vi "Extract zero offset.vi"(10 "Zero avg num":i32, 11 "Array":dbl[](array[numeric])) -> (3 "Offset":dbl)   [LabVIEW 2024]
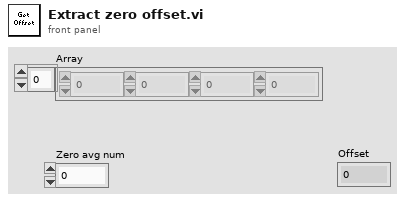
[diagram p1: front panel]
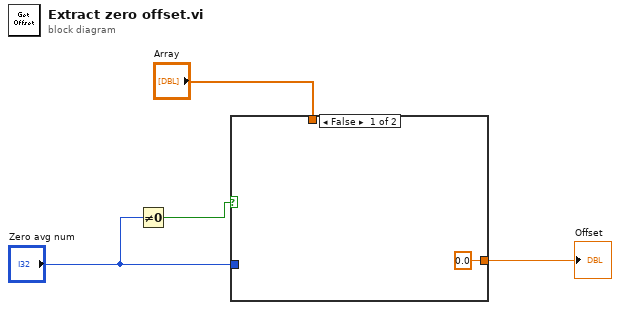
[diagram p0: block diagram]
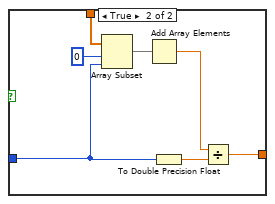
[diagram p2: hidden frame]
diagram:
  n1 = Not Equal To 0?(x="Zero avg num") -> (x != 0?=w1:bool)
  n2 = case shown="False" w1 {
    tunnel: "Array" -> [_ w12]
    tunnel: [0.0 w11] -> w3
    tunnel: "Zero avg num" -> [_ w9]
    frame False {
    }
    frame True {
      n3 = Array Subset(array=w12, index=0, length=w9) -> (w7:dbl[])
      n4 = Add Array Elements(numeric array=w7) -> (sum=w8:dbl)
      n5 = To Double Precision Float(number=w9) -> (double precision float=w10:dbl)
      n6 = Divide(x=w8, y=w10) -> (x/y=w11:dbl)
    }
  }
  "Offset" <- w3
